vi "Initialize Channel Group Commands Page.vi"(0 "channel group reference in":T1 format="%.0x", 11 "error in":errorcluster) -> (4 "channel group reference out":T1 format="%.0x", 15 "error out":errorcluster)   [LabVIEW 2019, in "Embedded Data Logger System Explorer.lvlib"]
uses:
  Embedded Data Logger System Explorer.lvlib
  <vilib>/NI VeriStand/Custom Device API/Custom Device API.lvlib
  <vilib>/NI VeriStand/Custom Device API/Custom Device Channel Type.ctl
  <vilib>/NI VeriStand/Custom Device API/Custom Device Channel.ctl
  Shared/Constants.vi
  Shared/Embedded Data Logger Shared.lvlib
  <vilib>/NI VeriStand/Custom Device API/Custom Device Item Ref.ctl
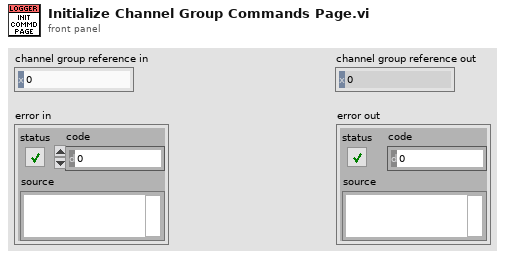
[diagram p1: front panel]
types:
  T1 = typedef "Custom Device API.lvlib/Custom Device Item Ref.ctl" = u64
  T2 = typedef "Custom Device API.lvlib/Custom Device Channel.ctl" = cluster{"Type":T3, "Units":string, "Default Value":dbl, "Faultable":bool, "Scalable":bool}
  T3 = typedef "Custom Device API.lvlib/Custom Device Channel Type.ctl" = enum16{"Input", "Output"}
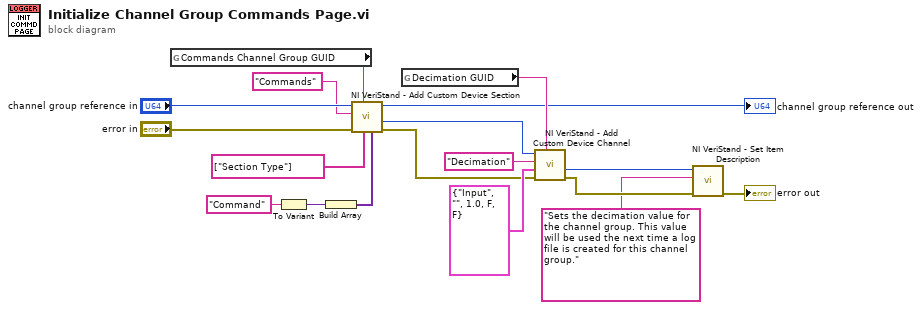
[diagram p0: block diagram]
diagram:
  n1 = global read "Constants.vi" "Commands Channel Group GUID"() -> (w12:string)
  n2 = To Variant(anything="Command" ("String")) -> (Variant=w4:variant)
  n3 = Build Array(w4) -> (w3:variant[])
  n4 = call <vilib>:"NI VeriStand - Add Custom Device Section.vi"("Property Values"=w3, "Property names"=string[] ["Section Type"], "GUID (Default Section)"=w12, "error in (no error)"="error in", "Section Name"="Commands", "Parent Ref in"="channel group reference in") -> ("error out"=w7:errorcluster, "Section Ptr"=w6:T1, "Parent Ref out"=→"channel group reference out":T1)  [unwired: 1 in, 2 out]
  n5 = global read "Constants.vi" "Decimation GUID"() -> (w11:string)
  n6 = call <vilib>:"NI VeriStand - Add Custom Device Channel.vi"("GUID (Default Channel)"=w11, "error in (no error)"=w7, "Channel"=T2 {"Type"=enum."Input", "Units"="", "Default Value"=1.0, "Faultable"=FALSE, "Scalable"=FALSE}, "Channel Name"="Decimation", "Parent Ref in"=w6) -> ("error out"=w14:errorcluster, "Channel Ref"=w13:T1)  [unwired: 3 in, 2 out]
  n7 = call <vilib>:"NI VeriStand - Set Item Description.vi"("error in (no error)"=w14, "Description"="Sets the decimation value for the channel group. This value will be used the next time a log file is created for this channel group." ("String"), "Item Ref in"=w13) -> ("error out"=→"error out":errorcluster)  [unwired: 6 in, 2 out]
